vi "Page_Source_Settings_Update_Display.vi"(6 "AB_Build in":refnum<class "AB_Build.lvclass">, 8 "error in (no error)":errorcluster, 9 "ctlReferences":T3, 10 "supportedFunctions":T2, 11 "AB_Source_Library in":refnum<class "AB_Source_Library.lvclass">) -> (0 "error out":errorcluster, 2 "parentApplies":T1, 3 "AB_Source_Library out":refnum<class "AB_Source_Library.lvclass">)   [LabVIEW 2020, in "AB_Source_Library.lvclass"]
uses:
  <vilib>/AppBuilder/AB_Classes/Source/Library/AB_Source_Library.lvclass
  e:/builds/penguin/labview/branches/2020/dev/dist/vi.lib/AppBuilder/AB_Classes/Source/AB_Source.lvclass
  <resource>/Framework/Providers/Builds/AppBuilder/AB_UI_Page_Source_Settings_References.ctl
  <resource>/Framework/Providers/Builds/AppBuilder/AB_UI_Page_Source_Settings_supportedFunctions.ctl
  <vilib>/AppBuilder/AB_Parent_Applies.ctl
  <vilib>/AppBuilder/AB_Classes/Build/AB_Build.lvclass
  <vilib>/AppBuilder/AB_Classes/Source/AB_Source.lvclass
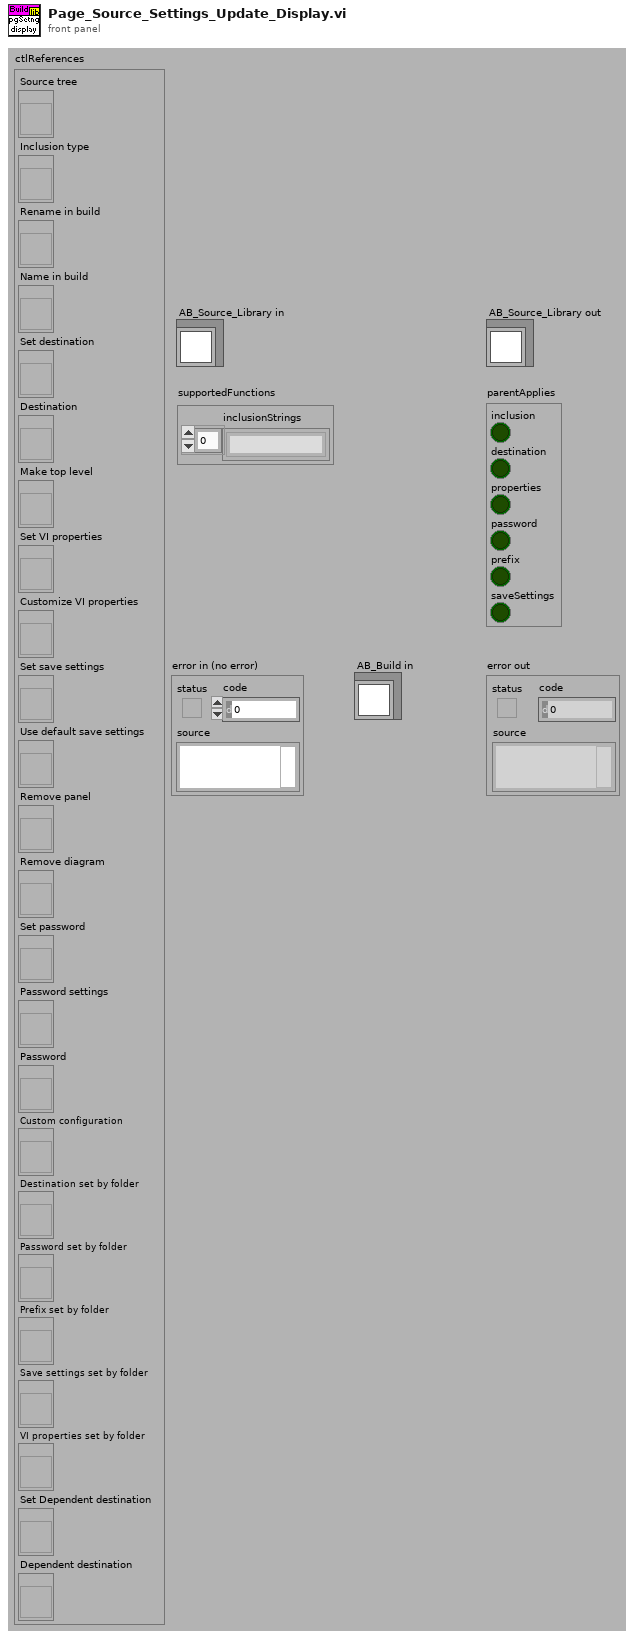
[diagram p1: front panel]
types:
  T1 = typedef "AB_Parent_Applies.ctl" = cluster{"inclusion":bool, "destination":bool, "properties":bool, "password":bool, "prefix":bool, "saveSettings":bool}
  T2 = typedef "AB_UI_Page_Source_Settings_supportedFunctions.ctl" = cluster{"inclusionStrings":string[]}
  T3 = typedef "AB_UI_Page_Source_Settings_References.ctl" = cluster{"Source tree":refnum<vi>, "Inclusion type":refnum<vi>, "Rename in build":refnum<vi>, "Name in build":refnum<vi>, "Set destination":refnum<vi>, "Destination":refnum<vi>, "Make top level":refnum<vi>, "Set VI properties":refnum<vi>, "Customize VI properties":refnum<vi>, "Set save settings":refnum<vi>, "Use default save settings":refnum<vi>, "Remove panel":refnum<vi>, "Remove diagram":refnum<vi>, "Set password":refnum<vi>, "Password settings":refnum<vi>, "Password":refnum<vi>, "Custom configuration":refnum<vi>, "Destination set by folder":refnum<vi>, "Password set by folder":refnum<vi>, "Prefix set by folder":refnum<vi>, "Save settings set by folder":refnum<vi>, "VI properties set by folder":refnum<vi>, "Set Dependent destination":refnum<vi>, "Dependent destination":refnum<vi>}
  T4 = typedef "AB_Source.ctl" = cluster{"path":path, "itemID":string, "parentIndex":i32, "sourceInclusion":T5, "destinationIndex":i32, "properties":T6[], "newName":string, "lvfile":bool, "valid":bool, "eng_inBuild":bool, "eng_isNonVILink":bool, "Amalgamation":bool, "Amalgamation Piece":bool, "eng_delimitedName":string, "preventRename":bool}
  T5 = typedef "AB_Source_Inclusion.ctl" = enum16{"IncludeIfReferenced", "Include", "Exclude", "TopLevel"}
  T6 = typedef "AB_Source_Properties.ctl" = cluster{"sourcePropertyType":T7, "value":variant}
  T7 = typedef "AB_Source_Property_Type.ctl" = enum16{"Remove block diagram", "Remove front panel", "Password", "Window has title bar", "Show menu bar", "Show vertical scroll bar", "Show horizontal scroll bar", "Show toolbar", "Show Abort button", "Show fp when called", "Window behavior", "Allow user to close window", "Window run-time position", "Run when opened", "Allow debugging", "Auto error handling", "Generate guard code", "Use stack variables", "Expression folding", "Integer only", "Inline subVI"}
  T8 = enum32{"No password change", "Remove password", "Apply new password"}
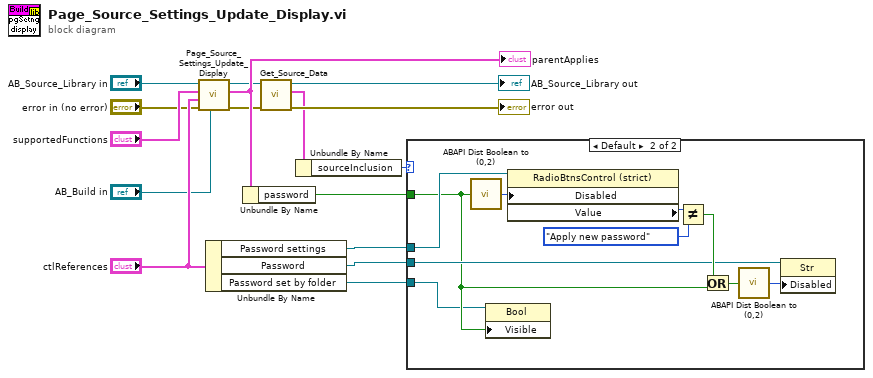
[diagram p0: block diagram]
diagram:
  n1 = call-parent "Page_Source_Settings_Update_Display.vi"("AB_Build in"="AB_Build in", "error in (no error)"="error in (no error)", "ctlReferences"="ctlReferences", "supportedFunctions"="supportedFunctions", "AB_Source in"="AB_Source_Library in") -> ("error out"=w6:errorcluster, "parentApplies"=w12:T1, "AB_Source out"=w8:refnum<class "AB_Source_Library.lvclass">)  [unwired: 4 in]
  "parentApplies" <- w12
  n2 = Unbundle By Name("ctlReferences") -> ("Password settings"=w14:refnum<vi>, "Password"=w13:refnum<vi>, "Password set by folder"=w1:refnum<vi>)
  n3 = Unbundle By Name(w12) -> ("password"=w11:bool)
  n4 = call <vilib>:"Get_Source_Data.vi"("error in (no error)"=w6, "Class in"=w8) -> ("error out"=→"error out":errorcluster, "data"=w4:T4, "Class out"=→"AB_Source_Library out":refnum<class "AB_Source_Library.lvclass">)  [unwired: 7 in]
  n5 = Unbundle By Name(w4) -> ("sourceInclusion"=w3:T5)
  n6 = case shown="Default" w3 {
    tunnel: w14 -> [_ w19]
    tunnel: w13 -> [_ w20]
    tunnel: w11 -> [_ w18]
    tunnel: w1 -> [_ w17]
    frame "Exclude" {
    }
    frame Default {
      n7 = call <vilib>:"ABAPI Dist Boolean to (0,2).vi"("Boolean"=w18) -> ("0, 2"=w21:u8)  [unwired: 4 in]
      n8 = property class="Bool"(reference=w17, "Visible"=w18) -> ()  [unwired: 1 in, 2 out]
      n9 = property class="RadioBtnsControl (strict)"(reference=w19, "Disabled"=w21) -> ("Value"=w26:T8)  [unwired: 1 in, 2 out]
      n10 = Not Equal?(x=w26, y=T8."Apply new password") -> (x != y?=w24:bool)
      n11 = Or(x=w24, y=w18) -> (x .or. y?=w23:bool)
      n12 = call <vilib>:"ABAPI Dist Boolean to (0,2).vi"("Boolean"=w23) -> ("0, 2"=w22:u8)  [unwired: 4 in]
      n13 = property class="Str"(reference=w20, "Disabled"=w22) -> ()  [unwired: 1 in, 2 out]
    }
  }
